vi "TE Signal2.0.vi"() -> ()   [LabVIEW 2010]
doc: "This example illustrates how to use autosetup and acquire multiple waveforms from several channels using the following steps:\n\n1. Specify a valid VISA session. \n2. Specify Channel A. \n3. Specify Channel B.\n4. Specify a time-out value for reading waveform.\n5. Run the VI. The graph displays waveforms you acquire."
uses:
  <vilib>/Platform/storage/lvStorage.llb/xStorage/Open Data Storage/Open Data Storage.xnode
  <vilib>/Platform/storage/lvStorage.llb/_openFunction.ctl
  <vilib>/Platform/storage/lvStorage.llb/xStorage/Set Properties/Set Properties.xnode
  <vilib>/Platform/storage/lvStorage.llb/xStorage/Write Data/Write Data.xnode
  <vilib>/Platform/storage/Storage.llb/usiOverwriteOptions.ctl
  <vilib>/Platform/storage/Storage.llb/usiSequenceRepresentation.ctl
  <vilib>/Platform/storage/lvStorage.llb/xStorage/Close Data Storage/Close Data Storage.xnode
  <instrlib>/Tektronix DPO MSO 2000 4000 Series/Public/Data/Read (Single Waveform).vi
  <instrlib>/Tektronix DPO MSO 2000 4000 Series/Public/Data/Read (Multiple Waveforms).vi
  <instrlib>/Tektronix DPO MSO 2000 4000 Series/Public/Configure/Configure Math (Dual).vi
  <vilib>/Platform/storage/lvStorage.llb/_openStorageWithRootAutoDetect.vi
  <vilib>/Platform/storage/lvStorage.llb/xStorage/xStorageSupp/ErrorOut.vi
  <vilib>/Platform/storage/Storage.llb/__savePropString.vi
  <vilib>/Platform/storage/Storage.llb/__savePropTime.vi
  <vilib>/Platform/storage/Storage.llb/_createExplicitChildObject.vi
  <vilib>/Platform/storage/lvStorage.llb/_prepDDT.vi
  <vilib>/Platform/storage/lvStorage.llb/_getChannelNameFromDDT.vi
  <vilib>/Platform/storage/lvStorage.llb/_saveDDT.vi
  <vilib>/Platform/storage/Storage.llb/Get Object Info.vi
  <vilib>/Platform/storage/Storage.llb/__closeStorageFromObject.vi
  <instrlib>/Tektronix DPO MSO 2000 4000 Series/Tektronix DPO MSO 2000 4000 Series.lvlib
panel:
  in  "Start TEST":bool
  out "?":bool
  out "?":bool
  out "DOWN":dbl
  out "UP":dbl
  in  "Error Range":dbl min=0.0 max=5.0 step=0.1 format="%#.3g"
  out "Pulse Duration":dbl
  out "TIMA":waveform(dbl)(graph)
  out "TIMB":waveform(dbl)(graph)
  out "Period":dbl
  in  "Assembled by":string="Alexis Ibarra"
  in  "ABM-S/N":string
  out "Differential Signal":waveform(dbl)(graph)
  in  "Port":u16(ring) items=["AMB 1", "AMB 2", "AMB 3", "AMB 4", "AMB 5", "AMB 18"]
  in  "DPO-4034 IP Adress":string
  out "error out":errorcluster
  in  "Maximum Time (10000ms)":u32=20000
  in  "Channel B (1: Channel 2)":u16(ring)=1 items=["Channel 1", "Channel 2", "Channel 3", "Channel 4", "Math", "Reference 1", "Reference 2", "Reference 3", "Reference 4"]
  in  "Channel A (0: Channel 1)":u16(ring) items=["Channel 1", "Channel 2", "Channel 3", "Channel 4", "Math", "Reference 1", "Reference 2", "Reference 3", "Reference 4"]
  out "TE Signals":waveform(dbl)[](graph)
  # "Actualy ip DPO-4038\n     10.195.18.178"
  # "Select Port"
  # "Error Limit"
  # "%"
  # "ms"
  # "ms"
  # "ms"
  # "Channels"
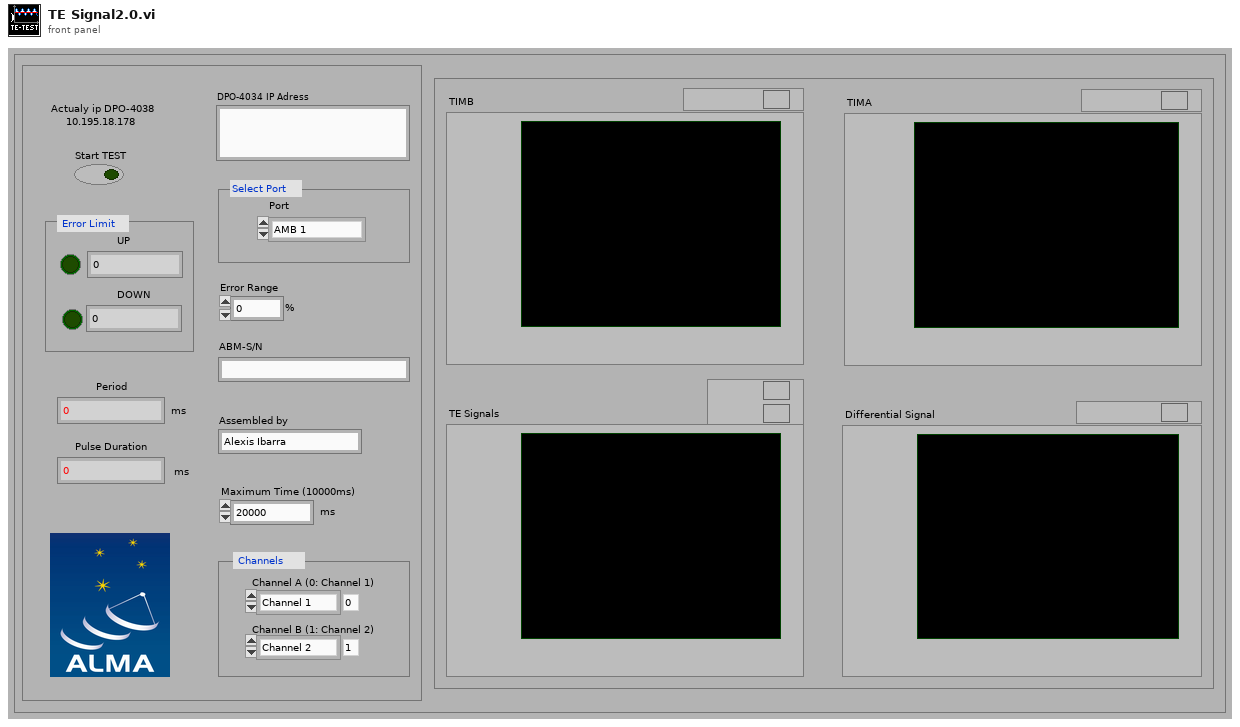
[diagram p1: front panel]
types:
  T1 = enum16{"UPDATE", "READ", "QUERY", "CREATE CHILD", "CREATE", "CONNECT", "DISCONNECT"}
  T2 = typedef "usiOverwriteOptions.ctl" = enum16{"Append values", "Replace values at index", "Replace all values", "Append if timeline aligns"}
  T3 = typedef "usiSequenceRepresentation.ctl" = enum16{"explicit", "implicit"}
  T4 = typedef "_openFunction.ctl" = enum16{"open", "open or create", "create or replace", "create", "open (read only)"}
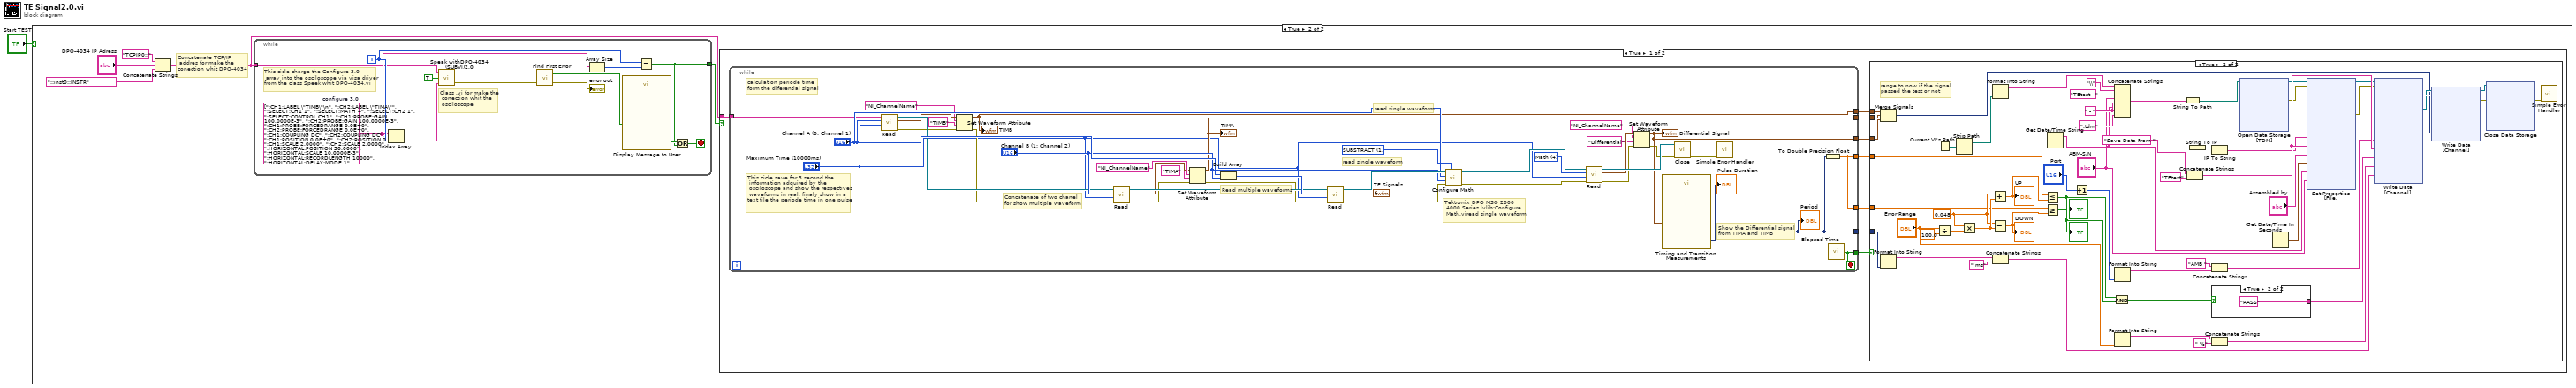
[diagram p0: block diagram]
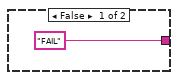
[diagram p4: hidden frame]
diagram:
  n1 = case shown="True" "Start TEST" {
    frame False {
    }
    frame True {
      # "Concatenate TCP/IP\n addres for make the \nconection whit DPO-4034"
      n2 = Concatenate Strings("TCPIP0::", "DPO-4034 IP Adress", "::inst0::INSTR") -> (w2:string)
      n3 = while {
        tunnel: w2 -> [w213]
        tunnel: [w210] -> w3
        i -> [w220]
        stop <- w215 stop-if-true
        w214 = string[] [":CH1:LABEL \"TIMB\"\n", ":CH2:LABEL \"TIMA\"", ":SELECT:CH1 1", ":SELECT:MATH 4", ":SELECT:CH2 1", ":SELECT:CONTROL CH1", ":CH1:PROBE:GAIN 100.0000E-3", ":CH2:PROBE:GAIN 100.0000E-3", ":CH1:PROBE:FORCEDRANGE 0.0E+0", ":CH2:PROBE:FORCEDRANGE 0.0E+0", ":CH1:COUPLING DC", ":CH2:COUPLING DC", ":CH1:POSITION 0.0E+0", ":CH2:POSITION 0.0E+0", ":CH1:SCALE 2.0000", ":CH2:SCALE 2.0000", ":HORIZONTAL:POSITION 50.0000", ":HORIZONTAL:SCALE 10.0000E-3", ":HORIZONTAL:RECORDLENGTH 10000", ":HORIZONTAL:DELAY:MODE 1", ":HORIZONTAL:DELAY:TIME 0.0E+0", ":TRIGGER:A:MODE AUTO", ":TRIGGER:A:TYPE EDGE", ":TRIGGER:A:LEVEL 2.0000", ":TRIGGER:A:LEVEL:CH2 2.0000", ":TRIGGER:A:UPPERTHRESHOLD:CH2 2.2000", ":TRIGGER:A:LOWERTHRESHOLD:CH2 2.000", ":TRIGGER:A:HOLDOFF:TIME 20.0000E-9", ":TRIGGER:A:EDGE:SOURCE CH2", ":TRIGGER:A:EDGE:COUPLING DC", ":TRIGGER:A:LOGIC:THRESHOLD:CH2 2.0000", ":TRIGGER:A:SETHOLD:DATA:SOURCE CH2", ":TRIGGER:A:SETHOLD:DATA:THRESHOLD 2.0000", ":ZOOM:GRATICULE:SIZE 80", ":DATA:SOURCE CH2", ":MATH:POSITION -3.00E-3", ":MATH:SCALE 2.0000"]  # configure 3.0
        # "Class .vi for make the\n conection whit the\n osciloscope"
        # "This cicle charge the Configure 3.0\n array into the osciloscope via visa driver \nfrom the class Speek whit DPO-4034.vi"
        n4 = Index Array "Index Array"(array=w214, index=w220) -> (element=w221:string)
        n5 = call "Speak withDPO-4034 (SUBVI)2.0.vi"("Send Command"=w221, "Send:  TRUE\nRecive: FALSE"=TRUE, "VISA Resource Name"=w213) -> ("error out"=w217:errorcluster)  [unwired: 1 out]
        n6 = call <vilib>:"Find First Error.vi"("error in (no error)"=w217) -> ("error out"=→"error out":errorcluster, "error?"=w211:bool)  [unwired: 3 in]
        n7 = Array Size(array=w214) -> (size(s)=w219:i32)
        n8 = call "Display Message to User"("Enable"=w211) -> ("OK"=w212:bool)  [unwired: 9 in, 1 out]
        n9 = Equal?(x=w220, y=w219) -> (x = y?=w210:bool)
        n10 = Or(x=w212, y=w210) -> (x .or. y?=w215:bool)
      }
      n11 = case shown="True" w3 {
        tunnel: w2 -> [w14 _]
        frame True {
          n12 = while {
            tunnel: [w182] -> w11
            tunnel: w14 -> [w197]
            tunnel: [w194] -> w13
            tunnel: [w186] -> w12
            tunnel: [w173] -> w8
            tunnel: [w174] -> w10
            tunnel: [w174] -> w9
            tunnel: [w172] -> w7
            stop <- w172 stop-if-true
            w175 = u16 4 items=["Channel 1", "Channel 2", "Channel 3", "Channel 4", "Math", "Reference 1", "Reference 2", "Reference 3", "Reference 4"] ("Channel (0: Channel 1)")
            w206 = u16 1 items=["ADD", "SUBSTRACT", "MULTIPLY", "DIVIDE"] ("Operator (0: ADD)")
            # "This cicle save for 3 second the\n information adquired by the\n osciloscope and show the respectives\n waveforms in real, finaly show in a \ntext file the periode time in one pulse"
            # "Concatenate of two chanel \nfor show multiple waveform"
            # "read single waveform"
            # "read single waveform"
            # "Tektronix DPO MSO 2000\n 4000 Series.lvlib:Configure\n Math.viread single waveform"
            # "calculation periode time\nform the diferential signal"
            # "Show the Differential signal \nfrom TIMA and TIMB"
            # "Read multiple waveforms"
            n13 = call-poly <instrlib>:"Read.vi"("Maximum Time (10000ms)"="Maximum Time (10000ms)", "Channel (0: Channel 1)"="Channel A (0: Channel 1)", "VISA resource name"=w197) -> ("error out"=w193:errorcluster, "Waveform Graph"=w196:waveform(dbl), "VISA resource name out"=w199:refnum<visa-resource-name>)  [unwired: 6 in]
            n14 = Set Waveform Attribute(4:w193, 5:"TIMB" ("name"), 6:"NI_ChannelName" ("name"), 7:w196) -> (0:w192:errorcluster, 3:w194:waveform(dbl))  [unwired: 1 out]
            "TIMB" <- w194
            n15 = call-poly <instrlib>:"Read.vi"("error in (no error)"=w192, "Maximum Time (10000ms)"="Maximum Time (10000ms)", "Channel (0: Channel 1)"="Channel B (1: Channel 2)", "VISA resource name"=w199) -> ("error out"=w188:errorcluster, "Waveform Graph"=w189:waveform(dbl), "VISA resource name out"=w198:refnum<visa-resource-name>)  [unwired: 5 in]
            n16 = Set Waveform Attribute(4:w188, 5:"TIMA" ("name"), 6:"NI_ChannelName" ("name"), 7:w189) -> (0:w187:errorcluster, 3:w186:waveform(dbl))  [unwired: 1 out]
            "TIMA" <- w186
            n17 = Build Array("Channel A (0: Channel 1)", "Channel B (1: Channel 2)") -> (w208:u16[])
            n18 = call-poly <instrlib>:"Read.vi"("error in (no error)"=w187, "Maximum Time (10000ms)"="Maximum Time (10000ms)", "Channels"=w208, "VISA resource name"=w198) -> ("error out"=w207:errorcluster, "Waveform Data"=→"TE Signals":waveform(dbl)[], "VISA resource name out"=w204:refnum<visa-resource-name>)  [unwired: 5 in]
            n19 = call-poly <instrlib>:"Configure Math.vi"("Operator (0: ADD)"=w206, "error in (no error)"=w207, "2nd Source (1: Channel 2)"="Channel B (1: Channel 2)", "1st Source (0: Channel 1)"="Channel A (0: Channel 1)", "VISA resource name"=w204) -> ("error out"=w203:errorcluster, "VISA resource name out"=w205:refnum<visa-resource-name>)  [unwired: 5 in]
            n20 = call-poly <instrlib>:"Read.vi"("error in (no error)"=w203, "Maximum Time (10000ms)"="Maximum Time (10000ms)", "Channel (0: Channel 1)"=w175, "VISA resource name"=w205) -> ("error out"=w181:errorcluster, "Waveform Graph"=w183:waveform(dbl), "VISA resource name out"=w202:refnum<visa-resource-name>)  [unwired: 5 in]
            n21 = Set Waveform Attribute(4:w181, 5:"Differential" ("name"), 6:"NI_ChannelName" ("name"), 7:w183) -> (0:w180:errorcluster, 3:w182:waveform(dbl))  [unwired: 1 out]
            "Differential Signal" <- w182
            n22 = call "Timing and Transition Measurements"("Signals"=w182) -> ("Period"=w173:dynamicdata, "Duration"=→"Pulse Duration":dynamicdata)  [unwired: 8 in, 1 out]
            "Period" <- w173
            n23 = call <instrlib>:"Close.vi"("error in (no error)"=w180, "VISA resource name"=w202) -> ("error out"=w209:errorcluster)  [unwired: 9 in]
            n24 = call <vilib>:"Simple Error Handler.vi"("error in (no error)"=w209) -> ()  [unwired: 4 in, 5 out]
            n25 = To Double Precision Float(number=w173) -> (double precision float=w174:dbl)
            n26 = call "Elapsed Time"() -> ("Time has Elapsed"=w172:bool)  [unwired: 12 in, 7 out]
          }
          n27 = case shown="True" w7 {
            tunnel: w13 -> [_ w20]
            tunnel: w12 -> [_ w19]
            tunnel: w11 -> [_ w18]
            tunnel: w10 -> [_ w17]
            tunnel: w9 -> [_ w16]
            tunnel: w8 -> [_ w15]
            frame False {
            }
            frame True {
              w47 = 0.048 ("x")
              w42 = " - " ("string")
              # "range to now if the signal\npassed the test or not"
              n28 = Merge Signals "Merge Signals"(w20, w19, w18) -> (w36:dynamicdata)
              n29 = Format Into String "Format Into String"(w15) -> (resulting string=w54:string)  [unwired: 3 in, 1 out]
              n30 = Divide(x="Error Range", y=100.0) -> (x/y=w46:dbl)
              n31 = Current VI's Path() -> (path=w27:path)
              n32 = Strip Path(path=w27) -> (stripped path=w26:path)  [unwired: 1 out]
              n33 = Multiply(x=w47, y=w46) -> (x*y=w48:dbl)
              n34 = Add(x=w47, y=w48) -> (x+y=w50:dbl)
              "UP" <- w50
              n35 = Subtract(x=w47, y=w48) -> (x-y=w51:dbl)
              "DOWN" <- w51
              n36 = Format Into String "Format Into String"(w26) -> (resulting string=w28:string)  [unwired: 3 in, 1 out]
              n37 = Concatenate Strings "Concatenate Strings"(w54, " ms") -> (w69:string)
              n38 = Less Or Equal?(x=w17, y=w50) -> (x <= y?=w52:bool)
              "?" <- w52
              n39 = Greater Or Equal?(x=w16, y=w51) -> (x >= y?=w53:bool)
              "?" <- w53
              n40 = Get Date/Time String() -> (date string=w41:string)  [unwired: 3 in, 1 out]
              n41 = Increment(x="Port") -> (x+1=w44:u16)
              n42 = And(x=w52, y=w53) -> (x .and. y?=w49:bool)
              n43 = Concatenate Strings "Concatenate Strings"(w28, "\\", "TEtest - " ("string"), "ABM-S/N", w42, w41, w42, ".tdm") -> (w24:string)
              n44 = Format Into String "Format Into String"(w44) -> (resulting string=w61:string)  [unwired: 3 in, 1 out]
              n45 = Format Into String "Format Into String"("Error Range") -> (resulting string=w57:string)  [unwired: 3 in, 1 out]
              n46 = String To Path(string=w24) -> (path=w23:path)
              n47 = Concatenate Strings "Concatenate Strings"("Save Data From ", "TEtest") -> (w70:string)
              n48 = String To IP() -> (0:w34:u32)  [unwired: 1 in]
              n49 = IP To String(2:w34) -> (0:w33:string)  [unwired: 1 in]
              n50 = Concatenate Strings "Concatenate Strings"("AMB ", w61) -> (w64:string)
              n51 = case shown="True" w49 {
                tunnel: ["FAIL" "PASS"] -> w67
                frame False {
                }
                frame True {
                }
              }
              n52 = Concatenate Strings "Concatenate Strings"(w57, " %") -> (w68:string)
              n53 = xnode "Open Data Storage\n[TDM]"("file path"=w23) -> ("storage refnum (file)"=w30:refnum<k20>, "error out"=w60:errorcluster)  [unwired: 4 in, 1 out]
              n54 = Get Date/Time In Seconds() -> (seconds since 1Jan1904=w29:timestamp)
              n55 = xnode "Set Properties\n[File]"("Name"=w33, "Description"=w70, "Author"="Assembled by", "Time stamp"=w29, "Date"=w41, "ABM_SerialNumber"="ABM-S/N", "storage refnum (file)"=w30, "error in"=w60) -> ("storage refnum (file) out"=w62:refnum<k20>, "error out"=w63:errorcluster)
              n56 = xnode "Write Data\n[Channel]"("Name"=w64, "Description"=w70, "Status"=w67, "Error_Range"=w68, "Periode"=w69, "storage refnum (file)"=w62, "error in"=w63) -> ("error out"=w66:errorcluster, "storage refnum (channel group)"=w65:refnum<k20>)  [unwired: 1 out]
              n57 = xnode "Write Data\n[Channel]"("Signal"=w36, "storage refnum (channel group)"=w65, "error in"=w66) -> ("storage refnum (channel group) out"=w37:refnum<k20>, "error out"=w38:errorcluster)  [unwired: 2 in, 1 out]
              n58 = xnode "Close Data Storage\n"("storage refnum (channel group)"=w37, "error in (no error)"=w38) -> ("error out"=w35:errorcluster)  [unwired: 1 out]
              n59 = call <vilib>:"Simple Error Handler.vi"("error in (no error)"=w35) -> ()  [unwired: 1 in, 8 out]
            }
          }
        }
        frame False {
        }
      }
    }
  }
